vi "switch.vi"(1 "Array 2":bool[](array[boolean]), 2 "Array 4":dbl[](array[numeric])) -> (0 "Array Out 3":dbl[](array[numeric]) format="%0.2f")   [LabVIEW 2013]
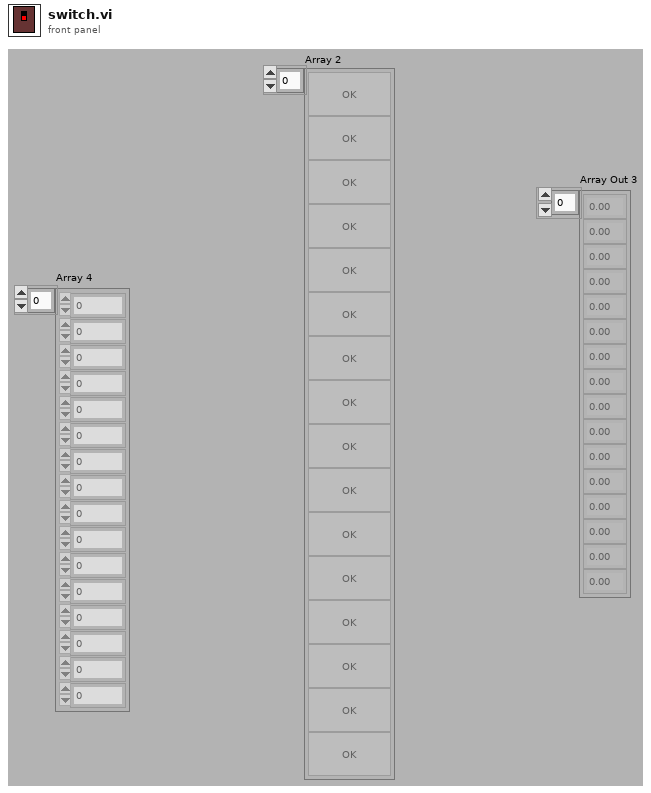
[diagram p1: front panel]
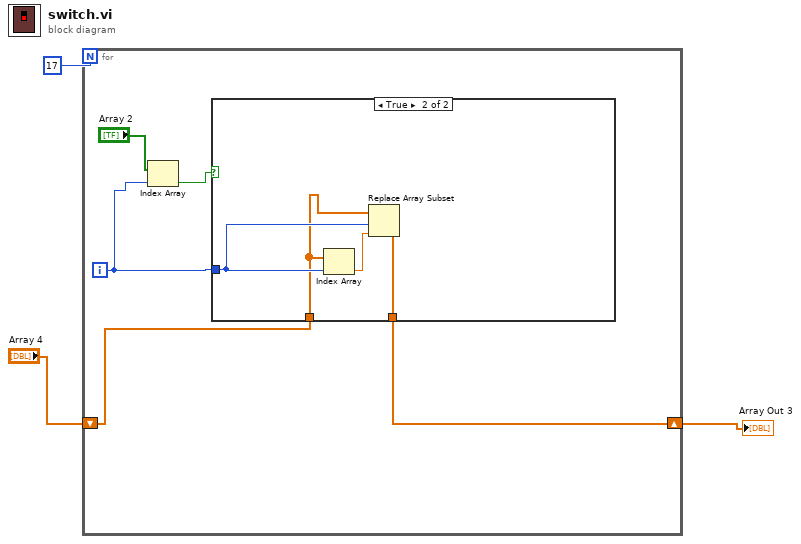
[diagram p0: block diagram]
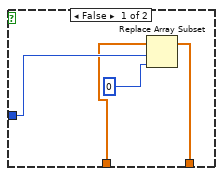
[diagram p2: hidden frame]
diagram:
  n1 = for {
    N: 17 -> [_]
    shift-right: [w4] -> w1
    shift-left: "Array 4" -> [w5]
    i -> [w8]
    n2 = Index Array(array="Array 2", index=w8) -> (element=w6:bool)
    n3 = case shown="True" w6 {
      tunnel: w8 -> [w12 w16]
      tunnel: w5 -> [w10 w14]
      tunnel: [w9 w13] -> w4
      frame False {
        n4 = Replace Array Subset(array=w10, new element=0, index=w12) -> (w9:dbl[])
      }
      frame True {
        n5 = Index Array(array=w14, index=w16) -> (element=w15:dbl)
        n6 = Replace Array Subset(array=w14, new element=w15, index=w16) -> (w13:dbl[])
      }
    }
  }
  "Array Out 3" <- w1
